vi "BagCollector-RT.vi"() -> ()   [LabVIEW 2014]
uses:
  Common/LaserScan.ctl
  <vilib>/robotics/TaimiOmni/TaimiOmni/TaimiOmniVelocity.ctl
  Common/Odometry.ctl
  Common/TwistCovariance.ctl
  <userlib>/ROS for LabVIEW Software/ROS/Code/Console/Servers/ServerSubs/TopicDef.ctl
  <userlib>/ROS for LabVIEW Software/ROS/Code/SubVIs/_ROSDirection.ctl
  <vilib>/myRIO/Instrument Drivers/Onboard IO/DIO/typedefs/DIO Reference.ctl
  <vilib>/myRIO/Common/Instrument Driver Framework/Utilities/typedefs/myRIO Generic Hardware Reference.ctl
  <vilib>/myRIO/Common/Instrument Driver Framework/Utilities/typedefs/Hardware Version Enum.ctl
  <vilib>/myRIO/Common/Instrument Driver Framework/Utilities/typedefs/myRIO v1.0 Reference.ctl
  <vilib>/myRIO/Common/Instrument Driver Framework/Utilities/typedefs/Generic FPGA Reference.ctl
  <vilib>/myRIO/Common/Instrument Driver Framework/myRIO v1.0/DIO/typedefs/DIO Channels List.ctl
  <vilib>/myRIO/Common/Instrument Driver Framework/myRIO v1.0/DIO/typedefs/DIO Channels Enum.ctl
  <vilib>/userdefined/High Color/nirio_resource_hc.ctl
  <vilib>/myRIO/Common/Instrument Driver Framework/Utilities/vis/Is FPGA Ref Available.vi
  <vilib>/myRIO/Common/Instrument Driver Framework/myRIO v1.0/DIO/vis/myRIO v1.1 Open DIO.vi
  <vilib>/myRIO/Instrument Drivers/Onboard IO/DIO/vis/Write.vi
  <vilib>/myRIO/Common/Instrument Driver Framework/Utilities/vis/Validate Channels.vi
  <vilib>/myRIO/Common/Instrument Driver Framework/myRIO v1.0/DIO/vis/myRIO v1.0 Reserve DIO.vi
  <vilib>/myRIO/Common/Instrument Driver Framework/myRIO v1.0/UART/vis/myRIO v1.0 Close UART.vi
  <vilib>/myRIO/Common/Instrument Driver Framework/myRIO v1.0/Resource Manager/vis/myRIO v1.0 Reserve Channel List.vi
  <vilib>/myRIO/Common/Instrument Driver Framework/myRIO v1.0/DIO/vis/myRIO v1.0 Build MUX Configuration DIO.vi
  <vilib>/myRIO/Common/Instrument Driver Framework/myRIO v1.0/Resource Manager/vis/myRIO v1.0 Reserve Channel.vi
  <vilib>/myRIO/Common/Instrument Driver Framework/myRIO v1.0/Resource Manager/vis/myRIO v1.0 Unreserve Channel.vi
  <vilib>/myRIO/Common/Instrument Driver Framework/myRIO v1.0/Resource Manager/vis/myRIO v1.0 Create Configuration List.vi
  <vilib>/myRIO/Common/Instrument Driver Framework/myRIO v1.0/Resource Manager/vis/myRIO v1.0 Build Mutex Name.vi
  <userlib>/ROS for LabVIEW Software/ROS/Code/_ROSDefinition.vi
  <instrlib>/Hokuyo URG Series/Public/Initialize-Standard.vi
  <vilib>/Utility/VariantDataType/GetNumericInfo.vi
  <vilib>/Utility/error.llb/Error Cluster From Error Code.vi
  <vilib>/myRIO/Common/Instrument Driver Framework/myRIO v1.0/myRIO v1.1 Open.vi
  <vilib>/myRIO/Common/Instrument Driver Framework/Utilities/vis/IO Manager.vi
  <vilib>/myRIO/Common/Instrument Driver Framework/Utilities/vis/Configuration Manager.vi
  <vilib>/myRIO/Common/Instrument Driver Framework/myRIO v1.0/Resource Manager/vis/myRIO v1.0 Configure IO.vi
  <vilib>/myRIO/Common/Instrument Driver Framework/myRIO v1.0/myRIO v1.0 Close.vi
  <vilib>/myRIO/Common/Instrument Driver Framework/myRIO v1.0/DIO/vis/myRIO v1.0 Write DIO.vi
  <vilib>/myRIO/Common/Instrument Driver Framework/Utilities/vis/FPGA Ref Manager.vi
  <vilib>/myRIO/Common/Instrument Driver Framework/myRIO v1.0/myRIO v1.0 Reset FPGA.vi
  <vilib>/myRIO/Common/Instrument Driver Framework/myRIO v1.0/IRQ/vis/myRIO v1.0 IRQ Info FGV.vi
  <vilib>/myRIO/Common/Instrument Driver Framework/myRIO v1.0/IRQ/vis/myRIO v1.0 Timer IRQ Info FGV.vi
  <vilib>/myRIO/Common/Instrument Driver Framework/myRIO v1.0/IRQ/vis/myRIO v1.0 ISR Agent.vi
  <vilib>/myRIO/Express VI/Onboard Devices/LED/LED Express VI.xnode
  <vilib>/myRIO/Instrument Drivers/Onboard IO/DIO/vis/myRIO DIO Open.xnode
  <vilib>/robotics/TaimiOmni/TaimiOmni (RT)/TaimiOmni (RT).lvclass
  <instrlib>/Hokuyo URG Series/Hokuyo URG Series.lvlib
  <vilib>/myRIO/Instrument Drivers/Onboard IO/DIO/DIO.lvlib
  <vilib>/myRIO/Instrument Drivers/Utilities/Utilities.lvlib
  <vilib>/robotics/TaimiOmni/TaimiOmni/TaimiOmni.lvclass
panel:
  out "OmniDynamics out":T1
  in  "odometry_frame":string="odometry"
  in  "base_link":string="base_link"
  in  "laser_frame_id":string="base_laser"
  out "TaimiOmniVelocity":T3
  in  "Y Velocity (m/s)":dbl(slide) min=-1.0 max=1.0 scale=-0.3..0.3
  in  "X Velocity (m/s)":dbl(slide) min=-1.0 max=1.0 scale=-0.3..0.3
  in  "Angular Velocity (rad/s)":dbl(slide) min=-2.0 max=2.0 scale=2.0..-2.0
  out "Y Velocity Feedback":dbl(slide) scale=-0.3..0.3
  out "X Velocity Feedback":dbl(slide) scale=-0.3..0.3
  out "Angular Velocity Feedback":dbl(slide) scale=2.0..-2.0
  in  "Breaked":bool
  in  "obstacle distance":dbl=0.12 format="%#_13g"
  in  "Stop":bool
  out "Data Aquired":picture
  in  "Grid Color":u32(colorbox)=16777222
  in  "Plot Color":u32(colorbox)=6618880
  in  "End Point":dbl=120.0
  in  "Start Point":dbl=-120.0
  in  "Cluster Count":dbl=1.0
  in  "Encoding Width":u16(ring)=3 items=["2 Byte"=2, "3 Byte"=3]
  in  "Max (m)":dbl=4.1
  out "LaserScan":T4
  in  "VISA resource name":refnum<visa-resource-name>
  in  "Checksum":bool
  in  "ID Query?":bool=TRUE
  in  "Protocol":u32(ring)=2 items=["Convert to Latest", "SCIP 1.1", "SCIP 2.0"]
  in  "polar attributes (hidden)":T5={"maximum"=30000.0, "minimum"=0.0, "clip to min"=FALSE, "log?(F)"=TRUE, "grid color"=6710886, "plot color"=65280, "fmt and prec"={"format"=enum."Decimal", "precision"=0}, "visible section"=8} {"minimum" format="%0.2f"; "maximum" format="%0.2f"}
  out "end":bool
  in  "ROS Master":string="172.16.0.10:11311"
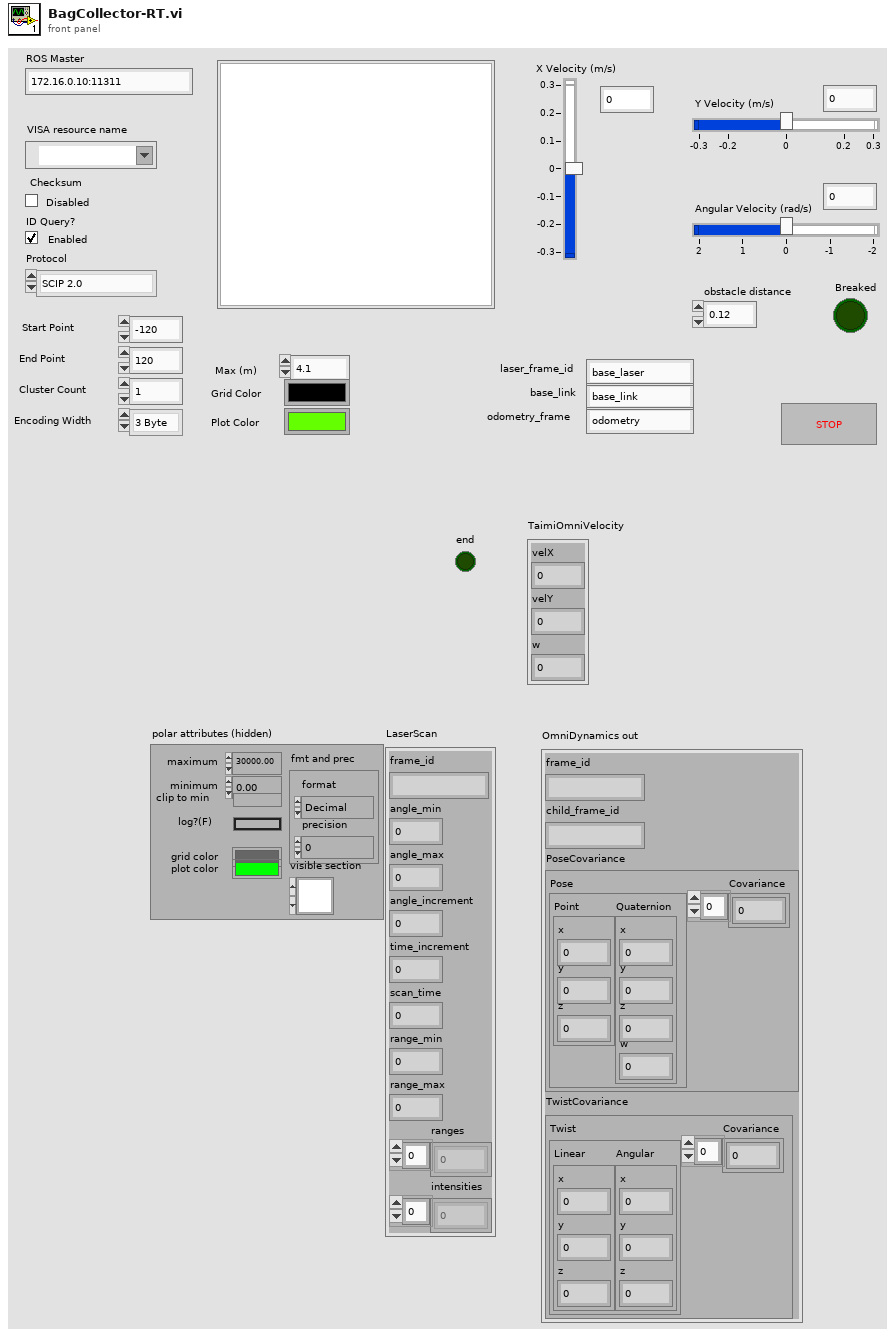
[diagram p1: front panel]
types:
  T1 = typedef "Odometry.ctl" = cluster{"frame_id":string, "child_frame_id":string, "PoseCovariance":cluster{"Pose":cluster{"Point":cluster{"x":dbl, "y":dbl, "z":dbl}, "Quaternion":cluster{"x":dbl, "y":dbl, "z":dbl, "w":dbl}}, "Covariance":dbl[]}, "TwistCovariance":T2}
  T2 = typedef "TwistCovariance.ctl" = cluster{"Twist":cluster{"Linear":cluster{"x":dbl, "y":dbl, "z":dbl}, "Angular":cluster{"x":dbl, "y":dbl, "z":dbl}}, "Covariance":dbl[]}
  T3 = typedef "TaimiOmni.lvclass/TaimiOmniVelocity.ctl" = cluster{"velX":dbl, "velY":dbl, "w":dbl}
  T4 = typedef "LaserScan.ctl" = cluster{"frame_id":string, "angle_min":dbl, "angle_max":dbl, "angle_increment":dbl, "time_increment":dbl, "scan_time":dbl, "range_min":dbl, "range_max":dbl, "ranges":dbl[], "intensities":dbl[]}
  T5 = cluster{"maximum":dbl, "minimum":dbl, "clip to min":bool, "log?(F)":bool, "grid color":u32, "plot color":u32, "fmt and prec":cluster{"format":enum8{"Decimal", "Scientific", "Engineering", "Binary", "Octal", "Hex"}, "precision":u8}, "visible section":u16}
  T6 = typedef "TopicDef.ctl" = cluster{"Topic":string, "Type":string, "Action":T7, "Update (ms)":u16, "queue size":u16}
  T7 = typedef "_ROSDirection.ctl" = enum16{"Node", "Publisher", "Subscriber", "ServiceClient", "ServiceProvider"}
  T8 = typedef "_ROSControl.ctl" = cluster{"topic port":u16, "Node":string, "topic":string, "type":string, "node port":u16, "error ":errorcluster, "Direction":T7, "Update (ms)":u16, "FIFO size":u16}
  T9 = typedef "DIO.lvlib/DIO Reference.ctl" = cluster{"myRIO Reference":T10, "DIO Channels List":T14}
  T10 = typedef "myRIO Generic Hardware Reference.ctl" = cluster{"myRIO Model":T11, "myRIO Hardware Reference":T12}
  T11 = typedef "Hardware Version Enum.ctl" = enum16{"Unknown", "myRIO-1900", "myRIO-1950"}
  T12 = typedef "myRIO v1.0 Reference.ctl" = cluster{"Generic FPGA Reference":T13, "Allow multiple opens":bool}
  T13 = typedef "Generic FPGA Reference.ctl" = refnum<k20>
  T14 = typedef "DIO Channels List.ctl" = T15[]
  T15 = typedef "DIO Channels Enum.ctl" = enum16{"Not Connected", "C/DIO0", "C/DIO1", "C/DIO2", "C/DIO3", "C/DIO4", "C/DIO5", "C/DIO6", "C/DIO7", "A/DIO0", "A/DIO1", "A/DIO2", "A/DIO3", "A/DIO4", "A/DIO5", "A/DIO6", "A/DIO7", "A/DIO8", "A/DIO9", "A/DIO10", "A/DIO11", "A/DIO12", "A/DIO13", "A/DIO14", "A/DIO15", "B/DIO0", "B/DIO1", "B/DIO2", "B/DIO3", "B/DIO4", "B/DIO5", "B/DIO6", "B/DIO7", "B/DIO8", "B/DIO9", "B/DIO10", "B/DIO11", "B/DIO12", "B/DIO13", "B/DIO14", "B/DIO15", "LED0", "LED1", "LED2", "LED3", "Button0"}
  T16 = typedef "nirio_resource_hc.ctl" = tag
  T17 = typedef "TaimiOmni.lvclass/TaimiOmniIRData.ctl" = cluster{"distance":dbl, "angle":dbl}
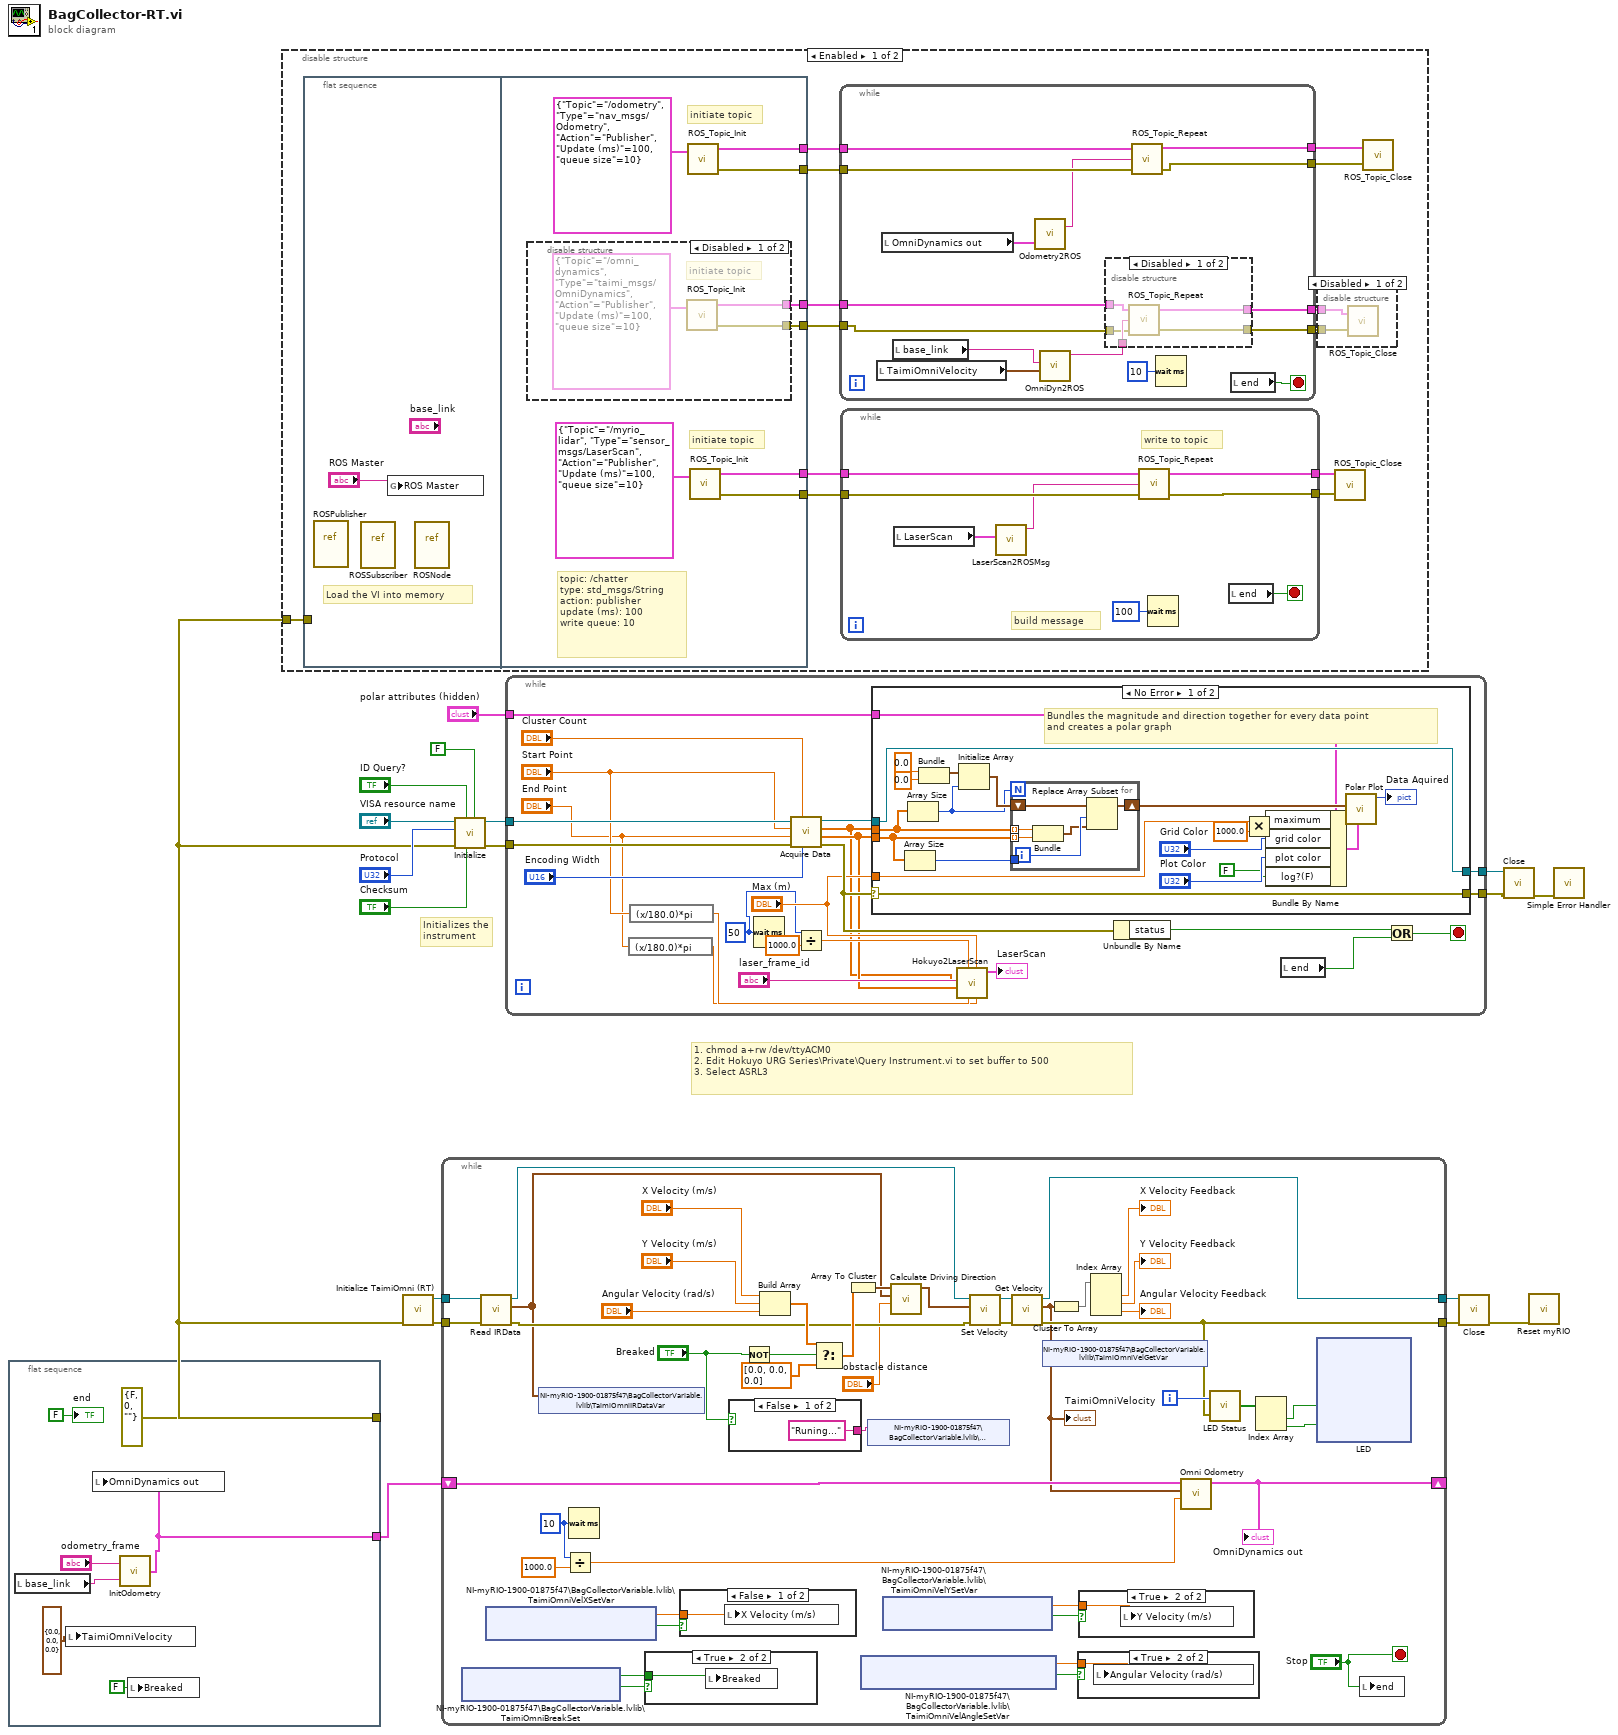
[diagram p0: block diagram]
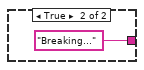
[diagram p6: hidden frame]
diagram:
  # "Initializes the instrument"
  # "1. chmod a+rw /dev/ttyACM0\n2. Edit Hokuyo URG Series\\Private\\Query Instrument.vi to set buffer to 500 \n3. Select ASRL3"
  n1 = flat-sequence {
    tunnel: [errorcluster {"status"=FALSE, "code"=0, "source"=""} ("error in (no error)")] -> w2
    tunnel: [w19] -> w1
    frame #0 {
      n2 = local read "base_link"() -> (w21:string)
      n3 = local write "TaimiOmniVelocity"(T3 {"velX"=0.0, "velY"=0.0, "w"=0.0} ("TaimiOmniVelocity")) -> ()
      n4 = call "InitOdometry.vi"("child_frame_id"=w21, "frame_id"="odometry_frame") -> ("OmniDynamics out"=w19:T1)
      n5 = local write "OmniDynamics out"(w19) -> ()
      n6 = local write "Breaked"(FALSE ("Breaked")) -> ()
      "end" <- FALSE ("end")
    }
  }
  n7 = disable-structure shown="Enabled" {
    disable-tunnel: w2 -> [w30 _]
    frame Enabled {
      n8 = flat-sequence {
        tunnel: w30 -> [_]
        tunnel: [w68] -> w38
        tunnel: [w67] -> w37
        tunnel: [w66] -> w34
        tunnel: [w65] -> w33
        tunnel: [w64] -> w32
        tunnel: [w63] -> w31
        frame #0 {
          # "Load the VI into memory"
          n9 = vi-ref <userlib>:"ROSPublisher.vi"() -> ()  [unwired: 1 out]
          n10 = vi-ref <userlib>:"ROSSubscriber.vi"() -> ()  [unwired: 1 out]
          n11 = global write "_ROSDefinition.vi" "ROS Master"("ROS Master") -> ()
          n12 = vi-ref <userlib>:"ROSNode.vi"() -> ()  [unwired: 1 out]
        }
        frame #1 {
          # "initiate topic"
          # "topic: /chatter\ntype: std_msgs/String\naction: publisher\nupdate (ms): 100\nwrite queue: 10"
          # "initiate topic"
          n13 = disable-structure shown="Disabled" {
            disable-tunnel: [w72 _] -> w66
            disable-tunnel: [w71 _] -> w65
            frame Disabled {
              # "initiate topic"
              n14 = call <userlib>:"ROS_Topic_Init.vi"("Definitions"=T6 {"Topic"="/omni_dynamics", "Type"="taimi_msgs/OmniDynamics", "Action"=enum."Publisher", "Update (ms)"=100, "queue size"=10}) -> ("ROS out"=w72:T8, "error out"=w71:errorcluster)  [unwired: 2 in]
            }
            frame Enabled {
            }
          }
          n15 = call <userlib>:"ROS_Topic_Init.vi"("Definitions"=T6 {"Topic"="/odometry", "Type"="nav_msgs/Odometry", "Action"=enum."Publisher", "Update (ms)"=100, "queue size"=10}) -> ("ROS out"=w64:T8, "error out"=w63:errorcluster)  [unwired: 2 in]
          n16 = call <userlib>:"ROS_Topic_Init.vi"("Definitions"=T6 {"Topic"="/myrio_lidar", "Type"="sensor_msgs/LaserScan", "Action"=enum."Publisher", "Update (ms)"=100, "queue size"=10}) -> ("ROS out"=w68:T8, "error out"=w67:errorcluster)  [unwired: 2 in]
        }
      }
      n17 = while {
        tunnel: w34 -> [w54]
        tunnel: w33 -> [w52]
        tunnel: [w51] -> w29
        tunnel: [w50] -> w28
        tunnel: w32 -> [w46]
        tunnel: w31 -> [w45]
        tunnel: [w44] -> w27
        tunnel: [w43] -> w26
        stop <- w49 stop-if-true
        n18 = local read "TaimiOmniVelocity"() -> (w55:T3)
        n19 = local read "OmniDynamics out"() -> (w42:T1)
        n20 = local read "base_link"() -> (w47:string)
        n21 = call "Odometry2ROS.vi"("OmniDynamics out"=w42) -> ("msg out"=w41:string)  [unwired: 2 in]
        n22 = call "OmniDyn2ROS.vi"("omni_dyn"=w55, "frame_id"=w47) -> ("msg out"=w53:string)  [unwired: 9 in]
        n23 = disable-structure shown="Disabled" {
          disable-tunnel: w54 -> [w60 _]
          disable-tunnel: w53 -> [w59 _]
          disable-tunnel: w52 -> [w58 _]
          disable-tunnel: [w57 _] -> w51
          disable-tunnel: [w56 _] -> w50
          frame Disabled {
            n24 = call <userlib>:"ROS_Topic_Repeat.vi"("error in (no error)"=w58, "Msg in"=w59, "ROS in"=w60) -> ("error out"=w56:errorcluster, "ROS out"=w57:T8)  [unwired: 1 in]
          }
          frame Enabled {
          }
        }
        n25 = call <userlib>:"ROS_Topic_Repeat.vi"("error in (no error)"=w45, "Msg in"=w41, "ROS in"=w46) -> ("error out"=w43:errorcluster, "ROS out"=w44:T8)  [unwired: 1 in]
        n26 = Wait (ms)(milliseconds to wait=u32 10) -> ()  [unwired: 1 out]
        n27 = local read "end"() -> (w49:bool)
      }
      n28 = while {
        tunnel: w38 -> [w80]
        tunnel: w37 -> [w79]
        tunnel: [w78] -> w36
        tunnel: [w77] -> w35
        stop <- w76 stop-if-true
        # "build message"
        # "write to topic"
        n29 = local read "LaserScan"() -> (w75:T4)
        n30 = call "LaserScan2ROSMsg.vi"("LaserScan"=w75) -> ("msg out"=w74:string)  [unwired: 10 in]
        n31 = call <userlib>:"ROS_Topic_Repeat.vi"("error in (no error)"=w79, "Msg in"=w74, "ROS in"=w80) -> ("error out"=w77:errorcluster, "ROS out"=w78:T8)  [unwired: 1 in]
        n32 = Wait (ms)(milliseconds to wait=u32 100) -> ()  [unwired: 1 out]
        n33 = local read "end"() -> (w76:bool)
      }
      n34 = disable-structure shown="Disabled" {
        disable-tunnel: w29 -> [w40 _]
        disable-tunnel: w28 -> [w39 _]
        frame Disabled {
          n35 = call <userlib>:"ROS_Topic_Close.vi"("error in"=w39, "ROS in"=w40) -> ()  [unwired: 2 in, 1 out]
        }
        frame Enabled {
        }
      }
      n36 = call <userlib>:"ROS_Topic_Close.vi"("error in"=w35, "ROS in"=w36) -> ()  [unwired: 2 in, 1 out]
      n37 = call <userlib>:"ROS_Topic_Close.vi"("error in"=w26, "ROS in"=w27) -> ()  [unwired: 2 in, 1 out]
    }
    frame Disabled {
    }
  }
  n38 = call <vilib>:"Initialize TaimiOmni (RT).vi"("error in (no error)"=w2) -> ("error out"=w6:errorcluster, "TaimiOmni (RT) out"=w7:refnum<class "TaimiOmni (RT).lvclass">)  [unwired: 9 in]
  n39 = while {
    tunnel: w7 -> [w95]
    tunnel: w6 -> [w94]
    tunnel: [w115] -> w4
    tunnel: [w113] -> w5
    shift-right: [w86] -> _
    shift-left: w1 -> [w87]
    i -> [w114]
    stop <- "Stop" stop-if-true
    w85 = u32 10 ("milliseconds to wait")
    n40 = shared-variable "NI-myRIO-1900-01875f47\\BagCollectorVariable.lvlib\\TaimiOmniBreakSet"() -> (w106:bool, w107:bool)  [unwired: 2 in, 1 out]
    n41 = call-dynamic "Read IRData.vi"("error in (no error)"=w94, "TaimiOmni in"=w95) -> ("error out"=w93:errorcluster, "IRData"=w90:T17[], "TaimiOmni out"=w92:refnum<class "TaimiOmni (RT).lvclass">)  [unwired: 7 in]
    n42 = shared-variable "NI-myRIO-1900-01875f47\\BagCollectorVariable.lvlib\\TaimiOmniVelXSetVar"() -> (w108:dbl, w109:bool)  [unwired: 2 in, 1 out]
    n43 = shared-variable "NI-myRIO-1900-01875f47\\BagCollectorVariable.lvlib\\TaimiOmniIRDataVar"(w90) -> ()  [unwired: 1 in, 1 out]
    n44 = Divide(x=w85, y=1000.0) -> (x/y=w83:dbl)
    n45 = Wait (ms)(milliseconds to wait=w85) -> ()  [unwired: 1 out]
    n46 = case shown="True" w107 {
      tunnel: w106 -> [_ w127]
      frame False {
      }
      frame True {
        n47 = local write "Breaked"(w127) -> ()
      }
    }
    n48 = case shown="False" w109 {
      tunnel: w108 -> [w166 _]
      frame False {
        n49 = local write "X Velocity (m/s)"(w166) -> ()
      }
      frame True {
      }
    }
    n50 = case shown="False" "Breaked" {
      tunnel: ["Runing..." ("TaimiOmniStatus") "Breaking..." ("TaimiOmniStatus")] -> w100
      frame False {
      }
      frame True {
      }
    }
    n51 = Not(x="Breaked") -> (.not. x?=w105:bool)
    n52 = Build Array("X Velocity (m/s)", "Y Velocity (m/s)", "Angular Velocity (rad/s)") -> (w104:dbl[])
    n53 = Select(t=w104, s=w105, f=dbl[] [0.0, 0.0, 0.0] ("t")) -> (s? t:f=w102:dbl[])
    n54 = Array To Cluster(array=w102) -> (cluster=w91:cluster{"t[0]":dbl, "t[1]":dbl, "t[2]":dbl})
    n55 = shared-variable "NI-myRIO-1900-01875f47\\BagCollectorVariable.lvlib\\TaimiOmniVelAngleSetVar"() -> (w97:dbl, w96:bool)  [unwired: 2 in, 1 out]
    n56 = shared-variable "NI-myRIO-1900-01875f47\\BagCollectorVariable.lvlib\\TaimiOmniStatus"(w100) -> ()  [unwired: 1 in, 1 out]
    n57 = shared-variable "NI-myRIO-1900-01875f47\\BagCollectorVariable.lvlib\\TaimiOmniVelYSetVar"() -> (w99:dbl, w98:bool)  [unwired: 2 in, 1 out]
    n58 = call "Calculate Driving Direction.vi"("obstacle distance"="obstacle distance", "IRData"=w90, "velocity in"=w91) -> ("velocity out"=w82:T3)  [unwired: 8 in]
    n59 = call-dynamic "Set Velocity.vi"("error in (no error)"=w93, "TaimiOmniVelocity"=w82, "TaimiOmni in"=w92) -> ("error out"=w120:errorcluster, "TaimiOmni out"=w121:refnum<class "TaimiOmni (RT).lvclass">)  [unwired: 7 in]
    n60 = call-dynamic "Get Velocity.vi"("error in (no error)"=w120, "TaimiOmni in"=w121) -> ("error out"=w113:errorcluster, "TaimiOmniVelocity"=w81:T3, "TaimiOmni out"=w115:refnum<class "TaimiOmni (RT).lvclass">)  [unwired: 7 in]
    "TaimiOmniVelocity" <- w81
    n61 = shared-variable "NI-myRIO-1900-01875f47\\BagCollectorVariable.lvlib\\TaimiOmniVelGetVar"(w81) -> ()  [unwired: 1 in, 1 out]
    n62 = Cluster To Array(cluster=w81) -> (array=w119:dbl[])
    n63 = case shown="True" w96 {
      tunnel: w97 -> [_ w128]
      frame False {
      }
      frame True {
        n64 = local write "Angular Velocity (rad/s)"(w128) -> ()
      }
    }
    n65 = case shown="True" w98 {
      tunnel: w99 -> [_ w129]
      frame False {
      }
      frame True {
        n66 = local write "Y Velocity (m/s)"(w129) -> ()
      }
    }
    n67 = Index Array(array=w119) -> (element #1=→"X Velocity Feedback":dbl, element #2=→"Y Velocity Feedback":dbl, element #3=→"Angular Velocity Feedback":dbl)  [unwired: 3 in]
    n68 = call "Omni Odometry.vi"("dt"=w83, "TaimiOmniVelocity"=w81, "OmniDynamics in"=w87) -> ("OmniDynamics out"=w86:T1)  [unwired: 8 in]
    "OmniDynamics out" <- w86
    n69 = call "LED Status.vi"("error in (no error)"=w113, "Interation"=w114) -> ("LEDs"=w112:bool[])
    n70 = Index Array(array=w112) -> (element #1=w111:bool, element #2=w110:bool)  [unwired: 2 in]
    n71 = xnode "LED"("LED0"=w111, "LED1"=w110) -> ()  [unwired: 1 in, 1 out]
    n72 = local write "end"("Stop") -> ()
  }
  n73 = call-poly <instrlib>:"Initialize.vi"("Reset? (F: No)"=FALSE ("Reset Instrument (Disabled)"), "Checksum (Disabled)"="Checksum", "ID Query? (Enabled)"="ID Query?", "error in (no error)"=w2, "Protocol (2: SCIP 2.0)"="Protocol", "VISA resource name"="VISA resource name") -> ("error out"=w9:errorcluster, "VISA resource name out"=w10:refnum<visa-resource-name>)  [unwired: 4 in]
  n74 = while {
    tunnel: w10 -> [w184]
    tunnel: [w190] -> w18
    tunnel: [w189] -> w11
    tunnel: w9 -> [w183]
    tunnel: "polar attributes (hidden)" -> [w182]
    stop <- w180 stop-if-true
    w170 = u32 50 ("milliseconds to wait")
    n75 = expression code="(x/180.0)*pi" ("degrees to radians")("End Point") -> (w175:dbl)
    n76 = expression code="(x/180.0)*pi" ("degrees to radians")("Start Point") -> (w177:dbl)
    n77 = Wait (ms)(milliseconds to wait=w170) -> ()  [unwired: 1 out]
    n78 = call <instrlib>:"Acquire Data.vi"("Data Encoding Width (3 Byte)"="Encoding Width", "Cluster Count (1)"="Cluster Count", "error in (no error)"=w183, "End Point (120°)"="End Point", "Start Point (-120°)"="Start Point", "VISA resource name"=w184) -> ("error out"=w186:errorcluster, "Direction"=w169:dbl[], "Magnitude"=w168:dbl[], "VISA resource name out"=w187:refnum<visa-resource-name>)  [unwired: 2 in]
    n79 = Divide(x=w170, y=1000.0) -> (x/y=w173:dbl)
    n80 = case shown="No Error" w186 {
      selector: w186 -> [w208 w218]
      tunnel: [w208 w218] -> w190
      tunnel: w187 -> [w209 w217]
      tunnel: [w209 w217] -> w189
      tunnel: w168 -> [w203 _]
      tunnel: w169 -> [w193 _]
      tunnel: w182 -> [w199 _]
      tunnel: "Max (m)" -> [w191 _]
      frame No Error {
        # "Bundles the magnitude and direction together for every data point\nand creates a polar graph"
        n81 = Array Size(array=w193) -> (size(s)=w192:i32)
        n82 = Array Size(array=w203) -> (size(s)=w202:i32)
        n83 = Bundle(0.0, 0.0) -> (w205:cluster{dbl, dbl})  [unwired: 1 in]
        n84 = Initialize Array(w205, w202) -> (w204:cluster{dbl, dbl}[])
        n85 = for {
          N: w202 -> [_]
          shift-right: [w212] -> w201
          shift-left: w204 -> [w213]
          tunnel: w203 -> [w216] mode=indexing
          tunnel: w193 -> [w215] mode=indexing
          tunnel: w192 -> [_]
          i -> [w214]
          n86 = Bundle(w216, w215) -> (w211:cluster{dbl, dbl})  [unwired: 1 in]
          n87 = Replace Array Subset(array=w213, new element=w211, index=w214) -> (w212:cluster{dbl, dbl}[])
        }
        n88 = Multiply(x=w191, y=1000.0) -> (x*y=w195:dbl)
        n89 = Bundle By Name(cluster=w199, "maximum"=w195, "grid color"="Grid Color", "plot color"="Plot Color", "log?(F)"=FALSE) -> (w200:T5)
        n90 = call <vilib>:"Polar Plot.vi"("polar attributes"=w200, "data array [mag, phase (deg)]"=w201) -> ("new picture"=→"Data Aquired":picture)  [unwired: 9 in]
      }
      frame Error {
      }
    }
    n91 = call "Hokuyo2LaserScan.vi"("angle_max"=w175, "range_max"="Max (m)", "angle_min"=w177, "scan_time"=w173, "Direction"=w169, "Magnitude"=w168, "frame_id"="laser_frame_id") -> ("LaserScan"=→"LaserScan":T4)  [unwired: 4 in]
    n92 = Unbundle By Name(w186) -> ("status"=w188:bool)
    n93 = local read "end"() -> (w167:bool)
    n94 = Or(x=w188, y=w167) -> (x .or. y?=w180:bool)
  }
  n95 = call-dynamic <instrlib>:"Close.vi"("error in (no error)"=w5, "TaimiOmni in"=w4) -> ("error out"=w3:errorcluster)  [unwired: 9 in]
  n96 = call <instrlib>:"Close.vi"("error in (no error)"=w18, "VISA resource name"=w11) -> ("error out"=w15:errorcluster)  [unwired: 9 in]
  n97 = call <vilib>:"Reset myRIO.vi"("error in (no error)"=w3) -> ()  [unwired: 10 in, 1 out]
  n98 = call <vilib>:"Simple Error Handler.vi"("error in (no error)"=w15) -> ()  [unwired: 4 in, 5 out]
